vi "Autonomous.vi"   [LabVIEW 2018]
doc: "This VI starts when autonomous period begins, and will automatically be terminated when it ends. You can carry out timed or sensor driven operations directly to I/O or to subsystems without needing to return to the caller."
uses:
  Auton/Auton Kill Switch.vi
  <vilib>/Rock Robotics/WPI/DriverStation/WPI_DriverStationDerivedRobotMode.ctl
  <vilib>/Rock Robotics/Network Tables/NT Read String.vi
  Wrist/Implementation/Wrist Published Globals.vi
types:
  T1 = typedef "ADIS16470 Device Reference.ctl" = cluster{"DevStatus":errorcluster, "Hardware Config":T2, "End Calibration":refnum<notifier>, "Calibration Complete":refnum<notifier>, "Data FIFO":refnum<k33>, "Status FIFO":refnum<k33>, "Last Value Reference":refnum<data-value>, "Sychronous Process VI":T6, "Cmd FIFO":refnum<k33>}
  T2 = typedef "ADIS16470 Hardware Configuration.ctl" = cluster{"SPI Clock Rate (Hz)":dbl, "IMU SPI Mode (3)":T3, "IMU Reset Pin":T4, "IMU SPI Bus":T5, "IMU Data Ready Pin":T4}
  T3 = typedef "WPI_SPIMode.ctl" = enum16{"Mode 0 (Clk Idle Low,Sample on Leading)", "Mode 1 (Clk Idle Low,Sample on Trailing)", "Mode 2 (Clk Idle High,Sample on Leading)", "Mode 3 (Clk Idle High,Sample on Trailing)"}
  T4 = typedef "FPGA_DIOChannel.ctl" = enum8{"DIO 0", "DIO 1", "DIO 2", "DIO 3", "DIO 4", "DIO 5", "DIO 6", "DIO 7", "DIO 8", "DIO 9", "DIO MXP 0", "DIO MXP 1", "DIO MXP 2", "DIO MXP 3", "DIO MXP 4", "DIO MXP 5", "DIO MXP 6", "DIO MXP 7", "DIO MXP 8", "DIO MXP 9", "DIO MXP 10", "DIO MXP 11", "DIO MXP 12", "DIO MXP 13", "DIO MXP 14", "DIO MXP 15", "SPI Port CS1", "SPI Port CS2", "SPI Port CS3", "SPI Port MISO", "SPI Port MOSI", "Invalid"}
  T5 = typedef "spi_bus.ctl" = enum16{"SPI On-Board, CS0", "SPI On-Board, CS1", "SPI On-Board, CS2", "SPI On-Board, CS3", "SPI MXP", "Invalid"}
  T6 = typedef "ADIS16470 Process.ctl" = refnum<vi>
  T7 = typedef "ADIS16470 Status.ctl" = cluster{"Calibrated?":bool}
  T8 = typedef "Command Status Info.ctl" = cluster{"Name":string, "Status":T9, "notifier out":T10}
  T9 = typedef "Completion Status.ctl" = enum16{"Successful", "Aborted", "Incomplete"}
  T10 = typedef "Completion Notifier.ctl" = refnum<notifier>
  T11 = typedef "WPI_JoystickDevRef.ctl" = cluster{"Device":T12}
  T12 = typedef "WPI_JoystickDeviceEnum.ctl" = enum16{"USB 0", "USB 1", "USB 2", "USB 3", "USB 4", "USB 5"}
  T13 = typedef "WPI_DriverStationDerivedRobotMode.ctl" = enum16{"Init", "Execute", "Stop"}
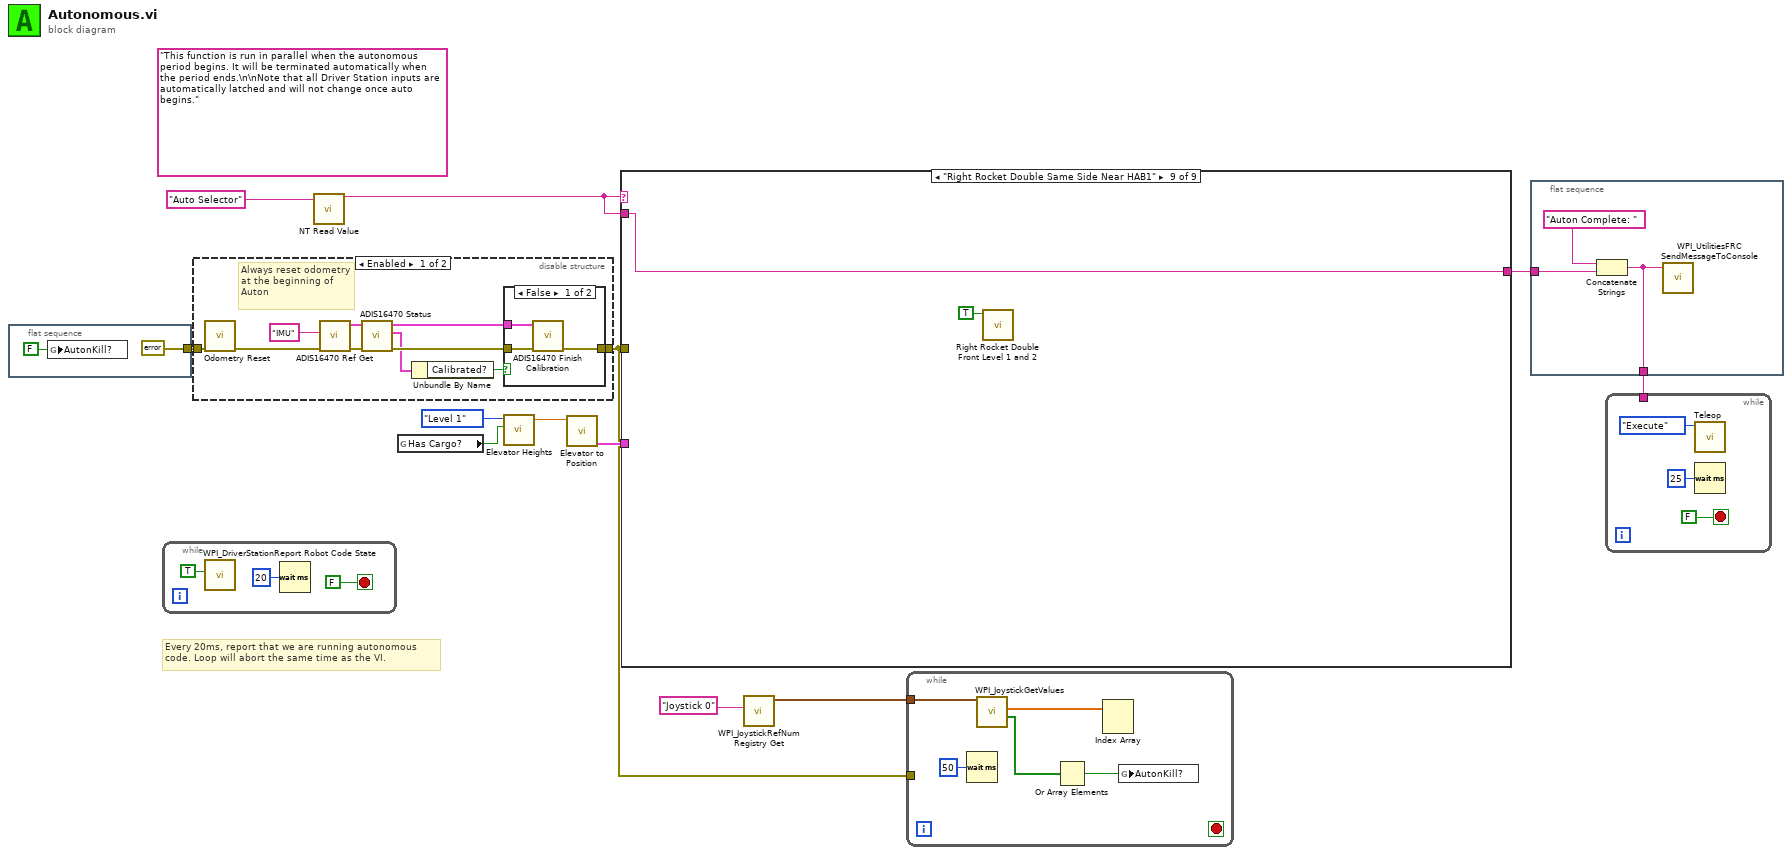
[diagram p0: block diagram]
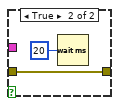
[diagram p2: hidden frame]
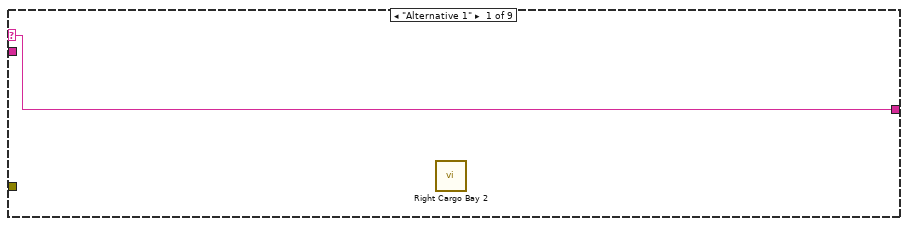
[diagram p4: hidden frame]
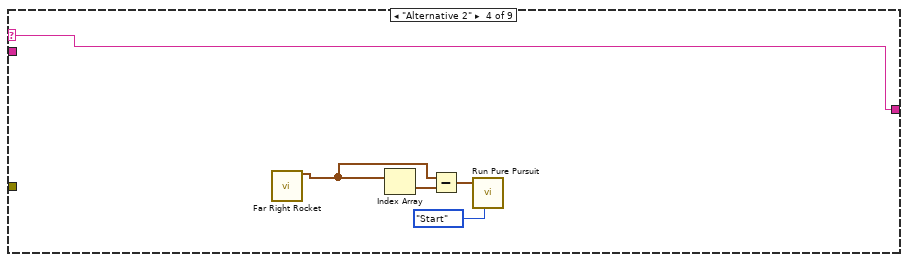
[diagram p7: hidden frame]
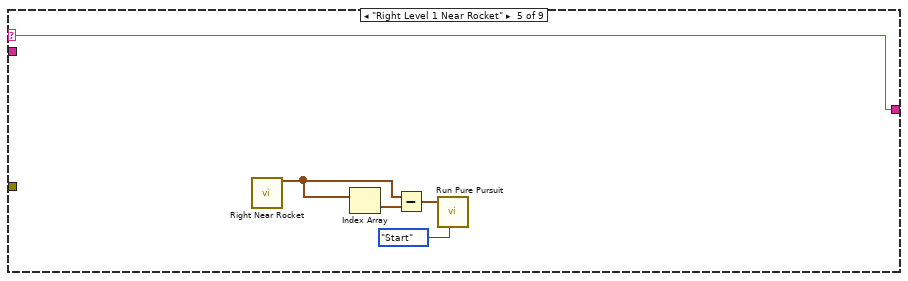
[diagram p8: hidden frame]
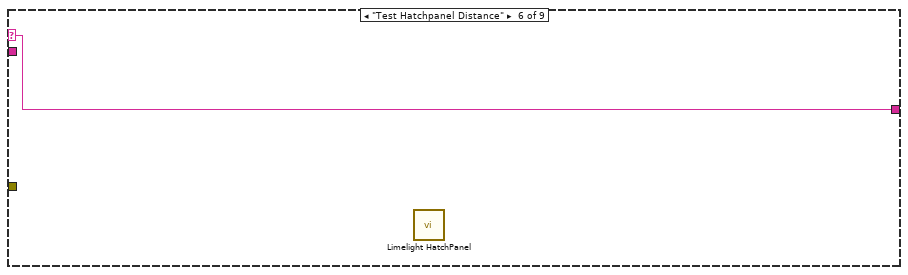
[diagram p9: hidden frame]
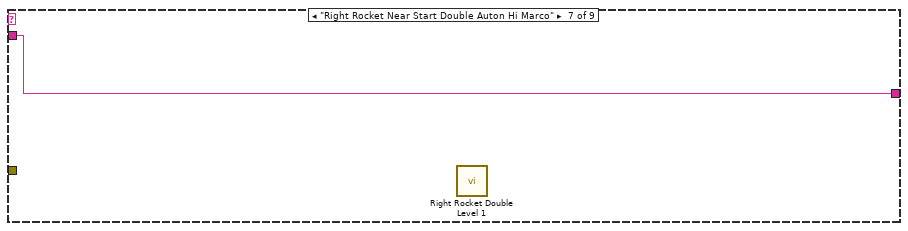
[diagram p10: hidden frame]
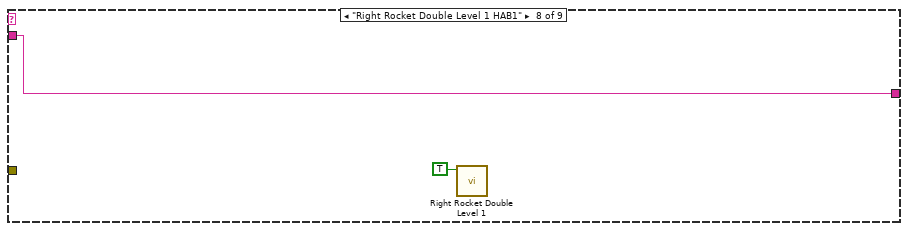
[diagram p11: hidden frame]
diagram:
  (unwired) "This function is run in parallel when the autonomous period begins. It will be terminated automatically when the period ends.\n\nNote that all Driver Station inputs are automatically latched and will not change once auto begins."
  # "Every 20ms, report that we are running autonomous\ncode. Loop will abort the same time as the VI."
  n1 = flat-sequence {
    tunnel: [errorcluster {"status"=FALSE, "code"=0, "source"=""} ("error in (no error)")] -> w9
    frame #0 {
      n2 = global write "Auton Kill Switch.vi" "AutonKill?"(FALSE ("AutonKill?")) -> ()
    }
  }
  n3 = while {
    stop <- FALSE stop-if-true
    n4 = call <vilib>:"WPI_DriverStationReport Robot Code State.vi"("Autonomous"=TRUE) -> ()  [unwired: 10 in, 1 out]
    n5 = Wait (ms)(milliseconds to wait=u32 20) -> ()  [unwired: 1 out]
  }
  n6 = disable-structure shown="Enabled" {
    disable-tunnel: [w27 _] -> w3
    disable-tunnel: w9 -> [w24 _]
    frame Enabled {
      # "Always reset odometry at the beginning of Auton"
      n7 = call "Odometry Reset.vi"("error in (no error)"=w24) -> ("error out"=w25:errorcluster)  [unwired: 10 in]
      n8 = call "ADIS16470 Ref Get.vi"("error in (no error)"=w25, "refnum name"="IMU") -> ("error out"=w23:errorcluster, "ADIS16470 Ref"=w20:T1)  [unwired: 8 in]
      n9 = call "ADIS16470 Status.vi"("error in (no error)"=w23, "ADIS16470DevRef"=w20) -> ("error out"=w22:errorcluster, "ADIS16470 Status"=w19:T7, "ADIS16470DevRef"=w21:T1)  [unwired: 7 in]
      n10 = Unbundle By Name(w19) -> ("Calibrated?"=w18:bool)
      n11 = case shown="False" w18 {
        tunnel: [w30 w32] -> w27
        tunnel: w22 -> [w29 w32]
        tunnel: w21 -> [w28 _]
        frame False {
          n12 = call "ADIS16470 Finish Calibration.vi"("error in (no error)"=w29, "ADIS16470DevRef in"=w28) -> ("error out"=w30:errorcluster)  [unwired: 8 in, 1 out]
        }
        frame True {
          n13 = Wait (ms)(milliseconds to wait=u32 20) -> ()  [unwired: 1 out]
        }
      }
    }
    frame Disabled {
    }
  }
  n14 = call-poly <vilib>:"NT Read Value.vi"("Name"="Auto Selector") -> ("String"=w4:string)  [unwired: 9 in, 1 out]
  n15 = global read "Wrist Published Globals.vi" "Has Cargo?"() -> (w5:bool)
  n16 = call "Elevator Heights.vi"("With Cargo?"=w5, "Level"=enum16{"Level 1", "Level 2", "Level 3"}."Level 1") -> ("Height"=w8:dbl)  [unwired: 7 in, 2 out]
  n17 = call "Elevator to Position.vi"("Elevator Height"=w8) -> ("Command Info Out"=w6:T8)  [unwired: 10 in]
  n18 = case shown="\"Right Rocket Double Same Side Near HAB1\"" w4 {
    selector: w4 -> [w33 w34 w35 w40 w41 w46 _ _ _]
    tunnel: w3 -> [_ _ _ _ _ _ _ _ _]
    tunnel: [w33 w34 w35 w40 w41 w46 w47 w49 w51] -> w11
    tunnel: w6 -> [_ _ _ _ _ _ _ _ _]
    tunnel: w4 -> [_ _ _ _ _ _ w47 w49 w51]
    frame "Alternative 1" {
      n19 = call "Right Cargo Bay 2.vi"() -> ()  [unwired: 12 in]
    }
    frame "Backup NT Auton" {
    }
    frame Default {
    }
    frame "Alternative 2" {
      n20 = call "Far Right Rocket.vi"() -> ("path"=w36:cluster{"X":dbl, "Y":dbl}[])  [unwired: 15 in]
      n21 = Index Array(array=w36) -> (element=w38:cluster{"X":dbl, "Y":dbl})  [unwired: 1 in]
      n22 = Subtract(x=w36, y=w38) -> (x-y=w37:cluster{"X":dbl, "Y":dbl}[])
      n23 = call "Run Pure Pursuit.vi"("Synchronication"=enum16{"Start", "Wait"}."Start", "Path"=w37) -> ()  [unwired: 9 in, 1 out]
    }
    frame "Right Level 1 Near Rocket" {
      n24 = call "Right Near Rocket.vi"() -> ("path"=w42:cluster{"X":dbl, "Y":dbl}[])  [unwired: 15 in]
      n25 = Index Array(array=w42) -> (element=w45:cluster{"X":dbl, "Y":dbl})  [unwired: 1 in]
      n26 = Subtract(x=w42, y=w45) -> (x-y=w44:cluster{"X":dbl, "Y":dbl}[])
      n27 = call "Run Pure Pursuit.vi"("Synchronication"=enum16{"Start", "Wait"}."Start", "Path"=w44) -> ()  [unwired: 9 in, 1 out]
    }
    frame "Test Hatchpanel Distance" {
      n28 = call "Limelight HatchPanel.vi"() -> ()  [unwired: 10 in, 2 out]
    }
    frame "Right Rocket Near Start Double Auton Hi Marco" {
      n29 = call "Right Rocket Double Level 1.vi"() -> ()  [unwired: 12 in]
    }
    frame "Right Rocket Double Level 1 HAB1" {
      n30 = call "Right Rocket Double Level 1.vi"("Level 1? (F)"=TRUE) -> ()  [unwired: 11 in]
    }
    frame "Right Rocket Double Same Side Near HAB1" {
      n31 = call "Right Rocket Double Front Level 1 and 2.vi"("Level 1? (F)"=TRUE) -> ()  [unwired: 11 in]
    }
  }
  n32 = call <vilib>:"WPI_JoystickRefNum Registry Get.vi"("refnum name"="Joystick 0") -> ("JoystickDevRef"=w1:T11)  [unwired: 1 in, 9 out]
  n33 = while {
    tunnel: w3 -> [_]
    tunnel: w1 -> [w56]
    stop <- _ stop-if-true
    n34 = Wait (ms)(milliseconds to wait=u32 50) -> ()  [unwired: 1 out]
    n35 = call <vilib>:"WPI_JoystickGetValues.vi"("JoystickDevRef"=w56) -> ("Buttons"=w54:bool[], "Axes"=w52:dbl[])  [unwired: 6 in, 3 out]
    n36 = Or Array Elements(Boolean array=w54) -> (logical OR=w53:bool)
    n37 = Index Array(array=w52) -> ()  [unwired: 2 in, 2 out]
    n38 = global write "Auton Kill Switch.vi" "AutonKill?"(w53) -> ()
  }
  n39 = flat-sequence {
    tunnel: w11 -> [w58]
    tunnel: [w57] -> w10
    frame #0 {
      n40 = Concatenate Strings("Auton Complete: " ("Message"), w58) -> (w57:string)
      n41 = call <vilib>:"WPI_UtilitiesFRC SendMessageToConsole.vi"("Message"=w57) -> ()  [unwired: 14 in, 1 out]
    }
  }
  n42 = while {
    tunnel: w10 -> [_]
    stop <- FALSE stop-if-true
    n43 = call "Teleop.vi"("Call Context"=WPI_DriverStationDerivedRobotMode."Execute") -> ()  [unwired: 11 in]
    n44 = Wait (ms)(milliseconds to wait=u32 25) -> ()  [unwired: 1 out]
  }
